vi "change titrant volume.vi"() -> (0 "incremental titrant added out":dbl format="%.2f")   [LabVIEW 2015]
panel:
  in  "OK Button":bool
  in  "incremental titrant added":dbl format="%.3f"
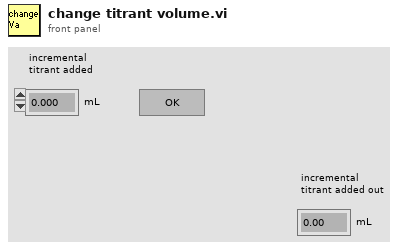
[diagram p1: front panel]
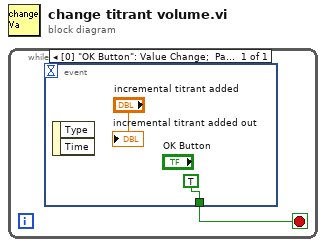
[diagram p0: block diagram]
diagram:
  n1 = while {
    stop <- w1 stop-if-true
    n2 = event shown="[0] \"OK Button\": Value Change;  Panel Close" {
      selector: _ -> [_]
      dyn-events: _ -> [_]
      timeout: _ -> [_]
      tunnel: [TRUE ("OK Button")] -> w1
      event "OK Button": Value Change; Panel Close {
        n3 = event-data() -> ()  [unwired: 1 in, 2 out]
        "incremental titrant added out" <- "incremental titrant added"
      }
    }
  }
